vi "Set Size.vi"(8 "error in (no error)":errorcluster, 10 "Size":cluster{"Width":i32, "Height":i32}, 11 "Drawer .Net in":refnum<class "Drawer .Net.lvclass">) -> (0 "error out":errorcluster, 3 "Drawer .Net out":refnum<class "Drawer .Net.lvclass">)   [LabVIEW 2020, in "Glyph .NET.lvlib" / "Drawer .Net.lvclass"]
uses:
  Drawer .Net.lvclass
  Drawer .Net.lvclass/Drawer .Net.ctl
  System.Drawing
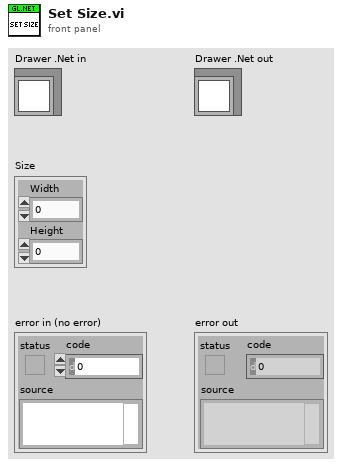
[diagram p1: front panel]
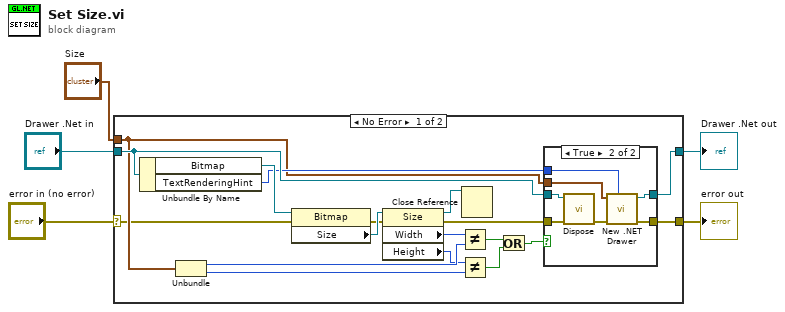
[diagram p0: block diagram]
diagram:
  n1 = case shown="No Error" "error in (no error)" {
    selector: "error in (no error)" -> [w8 w34]
    tunnel: [w12 w34] -> w4
    tunnel: [w11 w33] -> w2
    tunnel: "Drawer .Net in" -> [w15 w33]
    tunnel: "Size" -> [w13 _]
    frame No Error {
      n2 = Unbundle By Name(w15) -> ("Bitmap"=w23:refnum<k24>, "TextRenderingHint"=w14:i32)
      n3 = Unbundle(w13) -> ("Width"=w20:i32, "Height"=w18:i32)
      n4 = property class="Bitmap"(reference=w23, error in=w8) -> (error out=w7:errorcluster, "Size"=w22:refnum<k24>)  [unwired: 1 out]
      n5 = property class="Size"(reference=w22, error in=w7) -> (reference out=w9:refnum<k24>, error out=w6:errorcluster, "Width"=w21:i32, "Height"=w19:i32)
      n6 = Not Equal?(x=w21, y=w20) -> (x != y?=w17:bool)
      n7 = Not Equal?(x=w19, y=w18) -> (x != y?=w16:bool)
      n8 = Close Reference(reference=w9) -> ()  [unwired: 1 in, 1 out]
      n9 = Or(x=w17, y=w16) -> (x .or. y?=w10:bool)
      n10 = case shown="True" w10 {
        tunnel: w15 -> [w25 w32]
        tunnel: w14 -> [_ w31]
        tunnel: w13 -> [_ w30]
        tunnel: w6 -> [w24 w28]
        tunnel: [w24 w27] -> w12
        tunnel: [w25 w26] -> w11
        frame False {
        }
        frame True {
          n11 = call-dynamic "Dispose.vi"("error in (no error)"=w28, "Canvas in"=w32) -> ("error out"=w29:errorcluster)  [unwired: 9 in]
          n12 = call "New .NET Drawer.vi"("TextRenderingHint"=w31, "error in (no error)"=w29, "Size"=w30) -> ("error out"=w27:errorcluster, "Canvas out"=w26:refnum<class "Drawer .Net.lvclass">)  [unwired: 7 in]
        }
      }
    }
    frame Error {
    }
  }
  "error out" <- w4
  "Drawer .Net out" <- w2
